vi "neslab_coms_moose.vi"(6 "error in":errorcluster, 7 "byte array\n(in)":string[](array[string])=["CA", "00", "01", "00", "00", "FE"], 8 "Bytes to Read":u32=8, 9 "COM Port IN":refnum<visa-resource-name>="COM12") -> (0 "error out 2":errorcluster, 1 "byte array\n(out)":string[](array[string]), 2 "Serial Read":string, 3 "COM Port OUT":refnum<visa-resource-name>="COM12")   [LabVIEW 2010]
doc: "This subVI handles all of the direct serial communication with the Neslab, including:\n- initialization of the serial ports\n- conversion from Hex string to an unsigned byte string\n- the Serial Comminucation with the Neslab Device\n- converting from unsigned bytes to Hex strings\n- closing the serial communication"
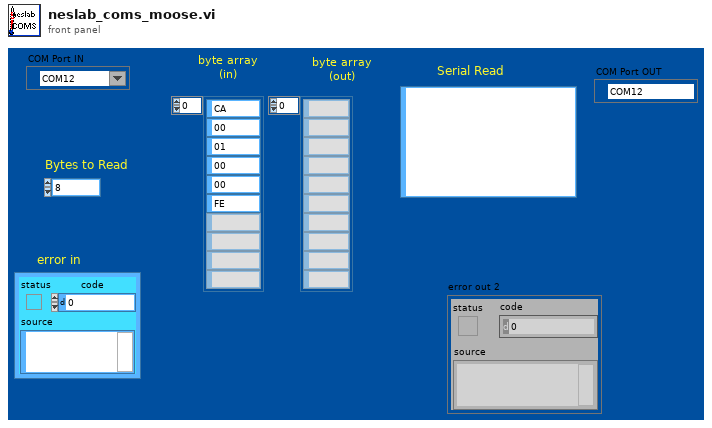
[diagram p1: front panel]
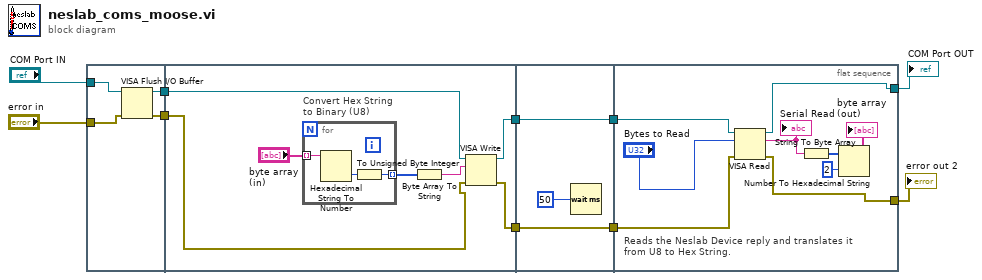
[diagram p0: block diagram]
diagram:
  n1 = flat-sequence {
    tunnel: "COM Port IN" -> [w14]
    tunnel: "error in" -> [w13]
    tunnel: [w12] -> w8
    tunnel: [w11] -> w7
    tunnel: [w16] -> w6
    tunnel: w8 -> [w18]
    tunnel: w7 -> [w17]
    tunnel: [w15] -> w3
    tunnel: w6 -> [w27]
    tunnel: [w27] -> w5
    tunnel: [w25] -> w4
    tunnel: w3 -> [w25]
    tunnel: w5 -> [w33]
    tunnel: w4 -> [w32]
    tunnel: [w29] -> w2
    tunnel: [w28] -> w1
    frame #0 {
      n2 = VISA Flush I/O Buffer(VISA resource name=w14, error in (no error)=w13) -> (VISA resource name out=w11:refnum<visa-resource-name>, error out=w12:errorcluster)  [unwired: 1 in]
    }
    frame #1 {
      # "Convert Hex String \nto Binary (U8)"
      n3 = for {
        tunnel: "byte array\n(in)" -> [w24] mode=indexing
        tunnel: [w22] -> w20 mode=indexing
        n4 = Hexadecimal String To Number(string=w24) -> (number=w23:u32)  [unwired: 2 in, 1 out]
        n5 = To Unsigned Byte Integer(number=w23) -> (unsigned 8bit integer=w22:u8)
      }
      n6 = Byte Array To String(unsigned byte array=w20) -> (string=w19:string)
      n7 = VISA Write(VISA resource name=w17, write buffer=w19, error in (no error)=w18) -> (VISA resource name out=w16:refnum<visa-resource-name>, error out=w15:errorcluster)  [unwired: 1 out]
    }
    frame #2 {
      n8 = Wait (ms)(milliseconds to wait=u32 50) -> ()  [unwired: 1 out]
    }
    frame #3 {
      # "Reads the Neslab Device reply and translates it\nfrom U8 to Hex String."
      n9 = VISA Read(VISA resource name=w33, byte count="Bytes to Read", error in (no error)=w32) -> (VISA resource name out=w28:refnum<visa-resource-name>, read buffer=w30:string, error out=w29:errorcluster)  [unwired: 1 out]
      "Serial Read" <- w30
      n10 = String To Byte Array(string=w30) -> (unsigned byte array=w35:u8[])
      n11 = Number To Hexadecimal String(1:2, 2:w35) -> (0:→"byte array\n(out)":string[])
    }
  }
  "error out 2" <- w2
  "COM Port OUT" <- w1
